vi "Configure Correction.vi"(8 "error in (no error)":errorcluster, 9 "Input Impedance Correction (0: 50 ohm)":i32(ring) items=["50 ohm", "75 ohm"], 10 "Enable Amplitude Correction (F: Disable)":bool, 11 "VISA resource name":refnum<visa-resource-name>) -> (0 "error out":errorcluster, 3 "VISA resource name out":refnum<visa-resource-name>)   [LabVIEW 2022 SP3, in "Agilent N934X Series.lvlib"]
doc: "Configure the amplitude correction function."
uses:
  <instrlib>/Agilent N934X Series/Agilent N934X Series.lvlib
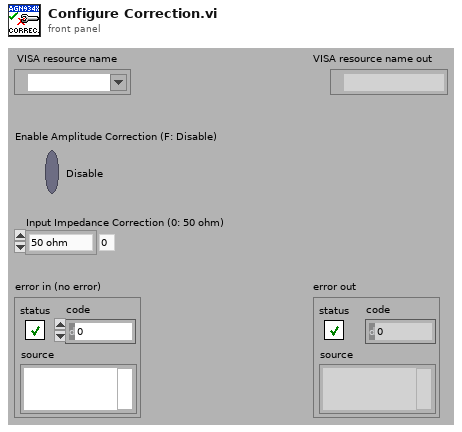
[diagram p1: front panel]
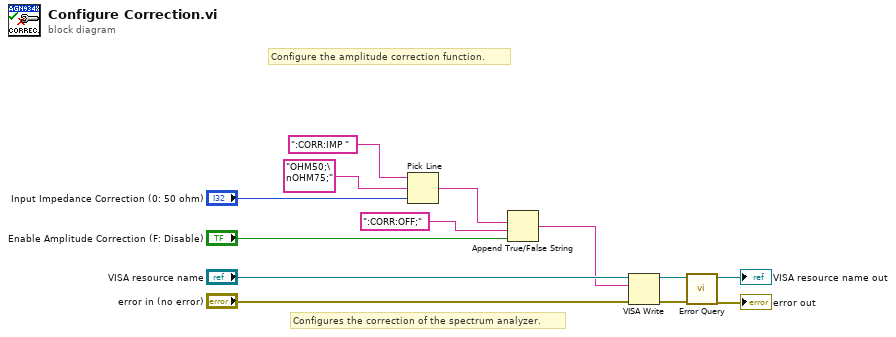
[diagram p0: block diagram]
diagram:
  # "Configures the correction of the spectrum analyzer."
  # "Configure the amplitude correction function."
  n1 = Pick Line(string ("")=":CORR:IMP ", multi-line string="OHM50;\nOHM75;", line index="Input Impedance Correction (0: 50 ohm)") -> (output string=w4:string)
  n2 = Append True/False String(1:"Enable Amplitude Correction (F: Disable)", 2:":CORR:OFF;", 3:w4) -> (0:w1:string)  [unwired: 1 in]
  n3 = VISA Write(VISA resource name="VISA resource name", write buffer=w1, error in (no error)="error in (no error)") -> (VISA resource name out=w11:refnum<visa-resource-name>, error out=w10:errorcluster)  [unwired: 1 out]
  n4 = call <instrlib>:"Error Query.vi"("error in (no error)"=w10, "VISA resource name"=w11) -> ("error out"=→"error out":errorcluster, "VISA resource name out"=→"VISA resource name out":refnum<visa-resource-name>)  [unwired: 6 in, 2 out]
